vi "Emballage_S0020002_TableauDonnees.vi"(8 "Indice Rev Client":string, 9 "N° article client":string, 10 "Chemin Logo":string, 11 "Tableau n° valves":string[](array[string])) -> (3 "Chaîne en sortie":string)   [LabVIEW 2020]
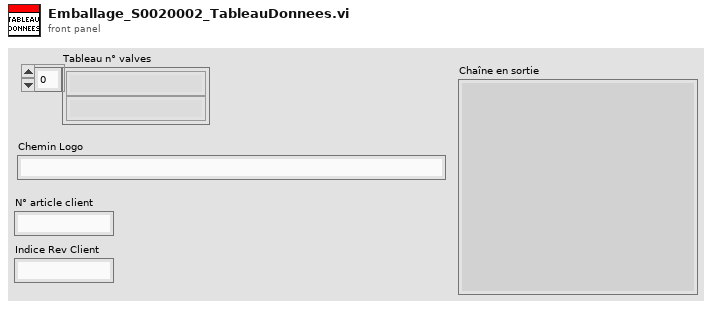
[diagram p1: front panel]
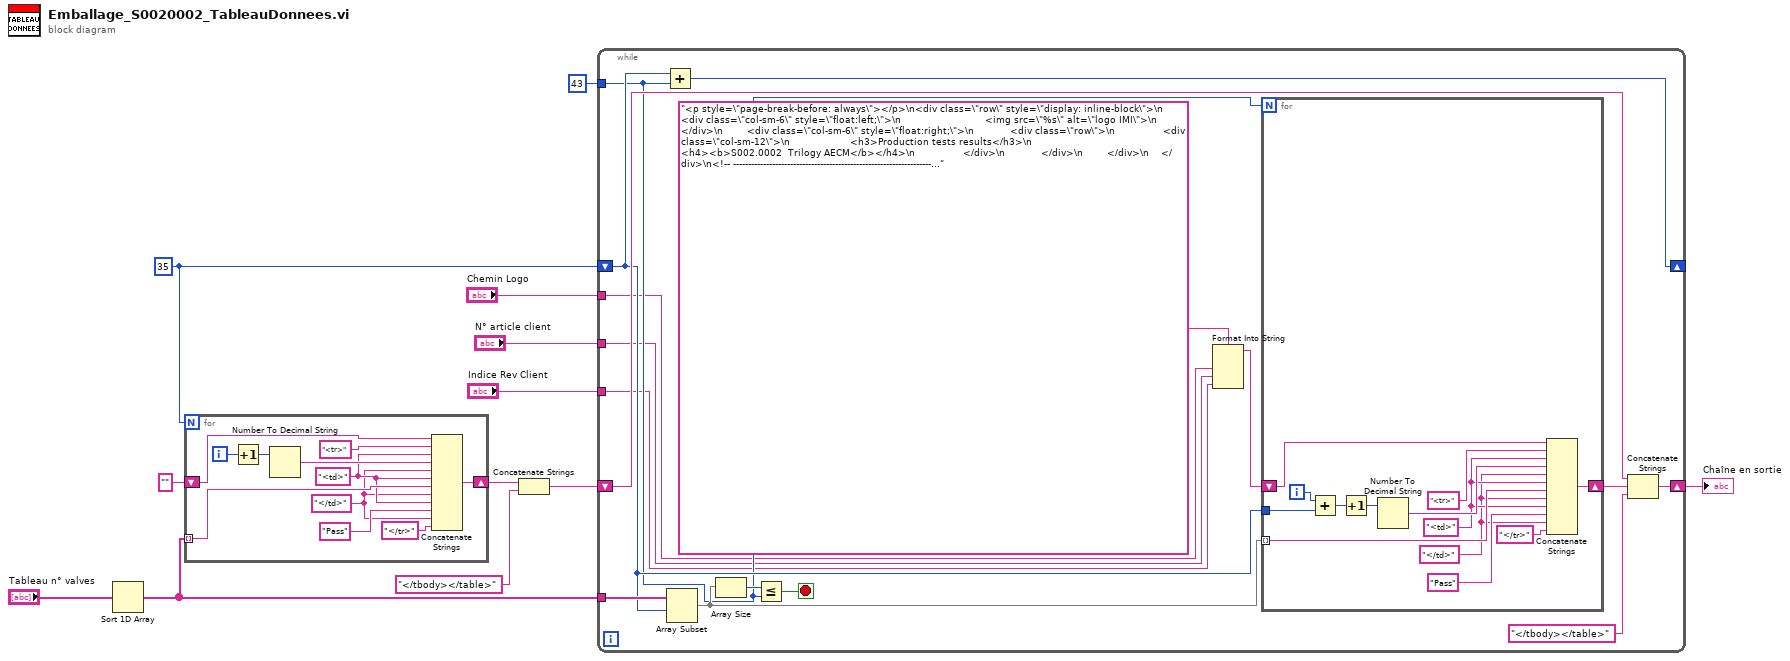
[diagram p0: block diagram]
diagram:
  w7 = 35
  n1 = Sort 1D Array(array="Tableau n° valves") -> (sorted array=w8:string[])
  n2 = for {
    N: w7 -> [_]
    tunnel: w8 -> [w17] mode=indexing
    shift-right: [w20] -> w5
    shift-left: "" -> [w21]
    i -> [w23]
    w14 = "</td>" ("chaîne")
    w16 = "<td>" ("chaîne")
    n3 = Increment(x=w23) -> (x+1=w22:i32)
    n4 = Number To Decimal String(number=w22) -> (decimal integer string=w18:string)  [unwired: 1 in]
    n5 = Concatenate Strings(w21, "<tr>" ("chaîne"), w16, w18, w14, w16, w17, w14, w16, "Pass" ("nouvel élément/sous-tableau"), w14, "</tr>" ("chaîne")) -> (w20:string)
  }
  n6 = Concatenate Strings(w5, "</tbody></table>") -> (w10:string)
  n7 = while {
    shift-right: [w35] -> w6
    shift-left: w10 -> [w36]
    tunnel: w8 -> [w34]
    shift-right: [w33] -> _
    shift-left: w7 -> [w32]
    tunnel: 43 -> [w29]
    tunnel: "Chemin Logo" -> [w26]
    tunnel: "N° article client" -> [w25]
    tunnel: "Indice Rev Client" -> [w24]
    stop <- w28 stop-if-true
    n8 = Add(x=w32, y=w29) -> (x+y=w33:i32)
    n9 = Array Subset(array=w34, index=w32) -> (w31:string[])  [unwired: 1 in]
    n10 = Array Size(array=w31) -> (size(s)=w30:i32)
    n11 = Less Or Equal?(x=w30, y=w29) -> (x <= y?=w28:bool)
    n12 = Format Into String(format string="<p style=\"page-break-before: always\"></p>\n<div class=\"row\" style=\"display: inline-block\">\n        <div class=\"col-sm-6\" style=\"float:left;\">\n                            <img src=\"%s\" alt=\"logo IMI\">\n                   </div>\n        <div class=\"col-sm-6\" style=\"float:right;\">\n            <div class=\"row\">\n                <div class=\"col-sm-12\">\n                    <h3>Production tests results</h3>\n                    <h4><b>S002.0002  Trilogy AECM</b></h4>\n                </div>\n            </div>\n        </div>\n    </div>\n<!-- ----------------------------------------------------------------------------------------- -->\n    <!-- Espace -->\n    <!-- ----------------------------------------------------------------------------------------- -->\n    <div class=\"row\">\n        <div class=\"col-sm-12\">\n            <br>\n                </div>\n    </div>\n<table><thead>\n                    <tr>\n                        <th></th>\n                        <th>Serial Number</th>\n                        <th>Test results according to<br>\n                            %s revision %s</th>\n                      </tr>\n                </thead><tbody>", w26, w25, w24) -> (resulting string=w27:string)  [unwired: 2 in, 1 out]
    n13 = for {
      N: w29 -> [_]
      tunnel: w31 -> [w46] mode=indexing
      shift-right: [w49] -> w38
      shift-left: w27 -> [w50]
      tunnel: w32 -> [w40]
      i -> [w52]
      w43 = "</td>" ("chaîne")
      w45 = "<td>" ("chaîne")
      n14 = Add(x=w52, y=w40) -> (x+y=w41:i32)
      n15 = Increment(x=w41) -> (x+1=w51:i32)
      n16 = Number To Decimal String(number=w51) -> (decimal integer string=w47:string)  [unwired: 1 in]
      n17 = Concatenate Strings(w50, "<tr>" ("chaîne"), w45, w47, w43, w45, w46, w43, w45, "Pass" ("nouvel élément/sous-tableau"), w43, "</tr>" ("chaîne")) -> (w49:string)
    }
    n18 = Concatenate Strings(w36, w38, "</tbody></table>") -> (w35:string)
  }
  "Chaîne en sortie" <- w6
